vi "Close_core.vi"(8 "error in (no error)":errorcluster, 11 "ctlrRef_VAT in":refnum<class "ctlRef_VAT.lvclass">) -> (0 "error out":errorcluster)   [LabVIEW 2020, in "CtlReferences.lvlib" / "ctlRef_VAT.lvclass"]
uses:
  ctlRef_VAT.lvclass
  CtlReferences/CtlReferences.lvclass
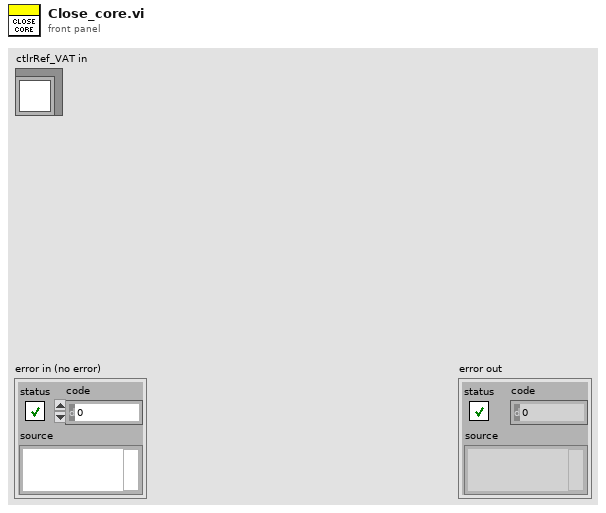
[diagram p1: front panel]
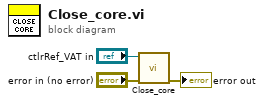
[diagram p0: block diagram]
diagram:
  n1 = call-parent "Close_core.vi"("error in (no error)"="error in (no error)", "CtlReferences in"="ctlrRef_VAT in") -> ("error out"=→"error out":errorcluster)  [unwired: 9 in]
